vi "Parthing And Build ResultString.vi"(11 "ResulIn":string[][](array[string])=[["ROI1_Numbers", "1"], ["ROI1_R_X_1", "287.75"], ["ROI1_R_Y_1", "-9.03"], ["ROI1_R_Angle_1", "-62.16"], ["ROI1_R_X_2", "0"], ["ROI1_R_Y_2", "0"], ["ROI1_R_Angle_2", "0"]]) -> (2 "ResultSend":string)   [LabVIEW 2019]
uses:
  e7aa767d-63a1-4d4e-8097-8e8619e10535.vi
  <vilib>/JDP Science/JSONtext/JSON text to Variant.vi
panel:
  out "Array 3":T1(array[cluster])
  out "Array 2":T2(array[cluster])
  out "Array":cluster{cluster{"ResultOut":string[][]}[]}[](array[cluster])
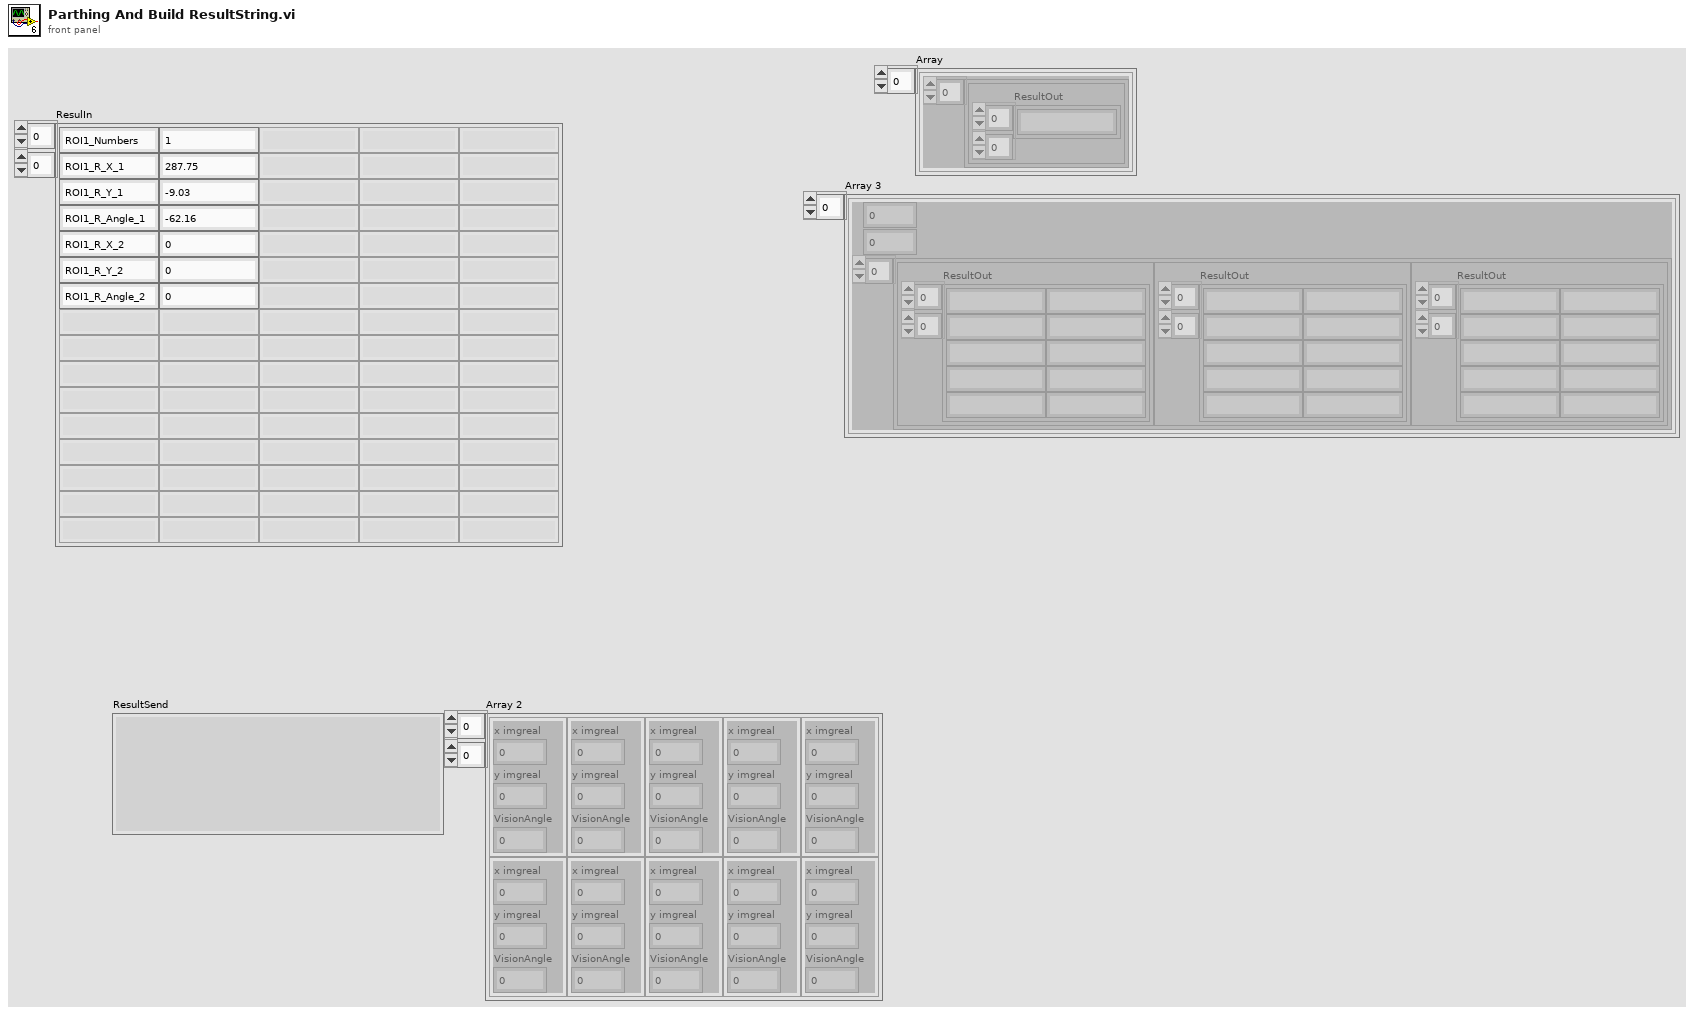
[diagram p1: front panel]
types:
  T1 = cluster{dbl, i32, cluster{"ResultOut":string[][]}[]}[]
  T2 = cluster{"x imgreal":dbl, "y imgreal":dbl, "VisionAngle":dbl}[][]
  T3 = enum16{"Initial", "Write", "Read", "Save", "Load", "WrteAll"}
  T4 = cluster{dbl, i32, cluster{"ResultOut":string[][]}[]}
  T5 = cluster{"x imgreal":dbl, "y imgreal":dbl, "VisionAngle":dbl}
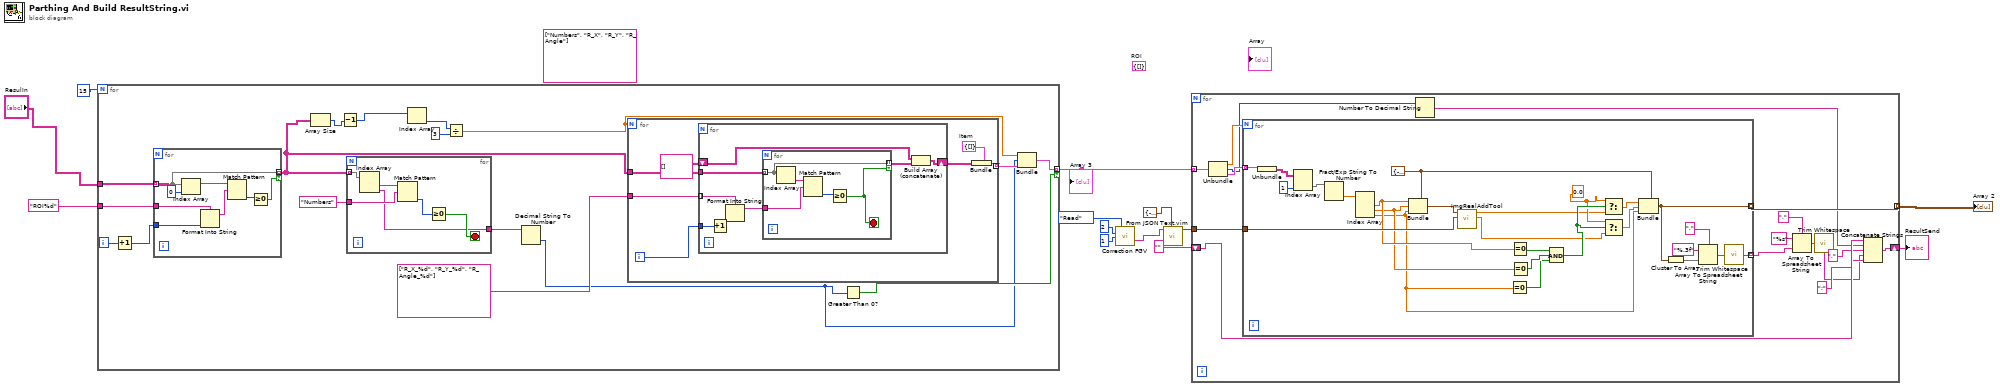
[diagram p0: block diagram]
diagram:
  (unwired) cluster{cluster{"ResultOut":string[][]}[]} {[]}  # ROI
  (unwired) string[] ["Numbers", "R_X", "R_Y", "R_Angle"]
  n1 = for {
    N: 15 -> [_]
    tunnel: "ResulIn" -> [w30]
    tunnel: "ROI%d" -> [w29]
    tunnel: [w22] -> w11 mode=indexing if=w21
    i -> [w28]
    n2 = Increment(x=w28) -> (x+1=w27:i32)
    n3 = for {
      tunnel: w30 -> [w58] mode=indexing
      tunnel: w29 -> [w62]
      tunnel: w27 -> [w61]
      tunnel: [w58] -> w19 mode=indexing if=w57
      n4 = Index Array(array=w58, index=0) -> (element=w64:string)
      n5 = Format Into String(format string=w62, w61) -> (resulting string=w60:string)  [unwired: 2 in, 1 out]
      n6 = Match Pattern(string=w64, regular expression=w60) -> (offset past match=w59:i32)  [unwired: 1 in, 3 out]
      n7 = Greater Or Equal To 0?(x=w59) -> (x >= 0?=w57:bool)
    }
    n8 = Array Size(array=w19) -> (size(s)=w18:i32[])
    n9 = Decrement(x=w18) -> (x-1=w17:i32[])
    n10 = for {
      tunnel: w19 -> [w36] mode=indexing
      tunnel: "Numbers" -> [w34]
      tunnel: [w31] -> w25
      stop <- w32 stop-if-true
      n11 = Index Array(array=w36) -> (element #1=w35:string, element #2=w31:string)  [unwired: 2 in]
      n12 = Match Pattern(string=w35, regular expression=w34) -> (offset past match=w33:i32)  [unwired: 1 in, 3 out]
      n13 = Greater Or Equal To 0?(x=w33) -> (x >= 0?=w32:bool)
    }
    n14 = Index Array(array=w17) -> (element=w16:i32)  [unwired: 1 in]
    n15 = Divide(x=w16, y=3) -> (x/y=w14:dbl)
    n16 = Decimal String To Number(string=w25) -> (number=w20:i32)  [unwired: 2 in, 1 out]
    n17 = for {
      N: w14 -> [_]
      tunnel: w19 -> [w43]
      tunnel: string[] ["R_X_%d", "R_Y_%d", "R_Angle_%d"] -> [w41]
      tunnel: [w38] -> w23 mode=indexing
      i -> [w42]
      w37 = cluster{"ResultOut":string[][]} {"ResultOut"=[]}  # Item
      n18 = for {
        tunnel: w43 -> [w51]
        tunnel: w42 -> [w50]
        tunnel: w41 -> [w49] mode=indexing
        shift-right: [w45] -> w39
        shift-left: string[][] [] ("ResultOut") -> [w44]
        n19 = Increment(x=w50) -> (x+1=w48:i32)
        n20 = Format Into String(format string=w49, w48) -> (resulting string=w47:string)  [unwired: 2 in, 1 out]
        n21 = for {
          tunnel: w51 -> [w53] mode=indexing
          tunnel: w47 -> [w54]
          tunnel: [w53] -> w46 mode=indexing if=w52
          stop <- w52 stop-if-true
          n22 = Index Array(array=w53) -> (element=w56:string)  [unwired: 1 in]
          n23 = Match Pattern(string=w56, regular expression=w54) -> (offset past match=w55:i32)  [unwired: 1 in, 3 out]
          n24 = Greater Or Equal To 0?(x=w55) -> (x >= 0?=w52:bool)
        }
        n25 = Build Array (concatenate)(w44, w46) -> (w45:string[][])
      }
      n26 = Bundle(cluster=w37, "ResultOut"=w39) -> (w38:cluster{"ResultOut":string[][]})
    }
    n27 = Greater Than 0?(x=w20) -> (x > 0?=w21:bool)
    n28 = Bundle(w14, w20, w23) -> (w22:T4)  [unwired: 1 in]
  }
  "Array 3" <- w11
  n29 = call "Correction FGV.vi"("Action"=T3."Read", "X"=2, "Y"=1) -> ("DataOut"=w7:string)  [unwired: 10 in, 2 out]
  n30 = call "From JSON Text.vim"("Data Type and Default Value"=cluster{"X":dbl, "Y":dbl, "Angle":dbl} {"X"=-45.8415, "Y"=-15.929499999999962, "Angle"=0.0} ("ToolData"), "JSON"=w7) -> ("Data out"=w5:cluster{"X":dbl, "Y":dbl, "Angle":dbl})  [unwired: 8 in, 1 out]
  n31 = for {
    tunnel: w11 -> [w80] mode=indexing
    tunnel: w5 -> [w79]
    tunnel: [w78] -> w4 mode=indexing
    shift-right: [w77] -> w2
    shift-left: "" -> [w76]
    n32 = Unbundle(w80) -> (w66:dbl, w65:i32, w67:cluster{"ResultOut":string[][]}[])
    n33 = for {
      N: w66 -> [_]
      tunnel: w67 -> [w106] mode=indexing
      tunnel: w79 -> [w100]
      tunnel: [w98] -> w78 mode=indexing
      tunnel: [w93] -> w73 mode=indexing
      w85 = 0.0
      w99 = T5 {"x imgreal"=-45.8415, "y imgreal"=-15.9295, "VisionAngle"=0.0} ("ImgRealData")
      n34 = Unbundle(w106) -> ("ResultOut"=w105:string[][])
      n35 = Index Array(array=w105, index (col)=1 ("disabled index (col)")) -> (element=w103:string[])  [unwired: 1 in]
      n36 = Fract/Exp String To Number(string=w103) -> (number=w102:dbl[])  [unwired: 3 in, 1 out]
      n37 = Index Array(array=w102) -> (element #1=w92:dbl, element #2=w91:dbl, element #3=w90:dbl)  [unwired: 3 in]
      n38 = Bundle(cluster=w99, "x imgreal"=w92, "y imgreal"=w91, "VisionAngle"=w90) -> (w101:T5)
      n39 = call "ImgRealAddTool.vi"("ToolData"=w100, "ImgRealData"=w101) -> ("YFinal"=w81:dbl, "XFinal"=w82:dbl)  [unwired: 8 in]
      n40 = Equal To 0?(x=w90) -> (x = 0?=w87:bool)
      n41 = Equal To 0?(x=w92) -> (x = 0?=w89:bool)
      n42 = Equal To 0?(x=w91) -> (x = 0?=w88:bool)
      n43 = Compound Arithmetic op=AND(w89, w88, w87) -> (w86:bool)
      n44 = Select(t=w85, s=w86, f=w82) -> (s? t:f=w84:dbl)
      n45 = Select(t=w85, s=w86, f=w81) -> (s? t:f=w83:dbl)
      n46 = Bundle(cluster=w99, "x imgreal"=w84, "y imgreal"=w83, "VisionAngle"=w90) -> (w98:T5)
      n47 = Cluster To Array(cluster=w98) -> (array=w97:dbl[])
      n48 = Array To Spreadsheet String(delimiter (Tab)=",", array=w97, 3:"%.3f" ("format string")) -> (spreadsheet string=w94:string)
      n49 = call <vilib>:"Trim Whitespace.vi"("string"=w94) -> ("trimmed string"=w93:string)  [unwired: 1 in]
    }
    n50 = Number To Decimal String(number=w65) -> (decimal integer string=w72:string)  [unwired: 1 in]
    n51 = Array To Spreadsheet String(delimiter (Tab)=",", array=w73, 3:"%s" ("format string")) -> (spreadsheet string=w70:string)
    n52 = call <vilib>:"Trim Whitespace.vi"("string"=w70) -> ("trimmed string"=w68:string)  [unwired: 1 in]
    n53 = Concatenate Strings(w76, w72, "," ("delimiter (Tab)"), w68, ";" ("delimiter (Tab)")) -> (w77:string)
  }
  "Array 2" <- w4
  "ResultSend" <- w2
